vi "Xml_Get_Version.vi"(8 "error in (no error)":errorcluster, 10 "XML Path":path=path "D:/TEST.xml", 11 "Refnum Cluster":refnum<vi>) -> (0 "error out":errorcluster, 3 "Version String":string)   [LabVIEW 2020]
doc: "This VI returns the XML version of a XML file.\nIf no XML version si found, returns an empty String."
uses:
  controls/EXPERT_Inputs.ctl
  controls/DIGIT_5122_Inputs.ctl
  <instrlib>/niScope/Controls/niScope trigger source.ctl
  controls/HSDIO_6541_Inputs.ctl
  <instrlib>/niHSDIO/niHSDIO.llb/niHSDIO_ctl Trigger Source Values (Ring).ctl
  controls/SOFTWARE_Inputs.ctl
  controls/AO_6711_Inputs.ctl
  controls/AWG_5421_Inputs.ctl
  <instrlib>/niFgen/niFgen.llb/niFgen_ctl Trigger Source Values (Ring).ctl
  controls/XML_Inputs.ctl
  <vilib>/NI/GXML/GXML.lvlib
panel:
  in  "EXPERT Inputs":T1={"DIGIT 5122 Inputs"={"Sample Rate"=10000.0, "Resource Name"="DIGIT_5122", "Channel Name"="0", "Trigger Source"="VAL_EXTERNAL", "Vertical Range"=10.0, "Trigger Level"=3.0}, "HSDIO 6541 Inputs"={"Resource Name"="HSDIO_6541", "Clock Rate"=1000000.0, "Trigger Source"="PFI0"}, "SOFTWARE Inputs"={"Application Directory"=path "D:/S.O.F.T.S/LABVIEW/PIL", "Software Version"="1.0.0", "Data Path"=path "D:/PIRENEA/DATA", "XML Path"=path "D:/PIRENEA/DATA", "XML File Filter"="*.xml", "XML Saved Path"=path "D:/PIRENEA/DATA/SAVED", "Excit Scripts Path"=path "D:/PIRENEA/EXCIT_SCRIPTS", "Excit Scripts File Filter"="*.txt", "Excit Waveforms Path"=path "D:/PIRENEA/EXCIT_WFMS", "Excit Waveforms File Filter"="*.bin", "Timing Scripts Path"=path "D:/PIRENEA/TIMING_SCRIPTS", "Timing Scripts File Filter"="*.txt", "Timing Waveforms Path"=path "D:/PIRENEA/TIMING_WFMS", "Timing Waveforms File Filter"="*.bin", "Trapping Waveforms Path"=path "D:/PIRENEA/TRAPPING_WFMS", "Trapping Waveforms File Filter"="*.bin"}, "AO 6711 Inputs"={"Physical Channels"="AO_6711/ao0:3", "Min Voltage"=-10.0, "Max Voltage"=10.0, "Trigger Source"="/AO_6711/PFI3", "Counter"="AO_6711/ctr0"}, "AWG 5421 Inputs"={"Resource Name"="AWG_5421", "Sample Rate"=10000000.0, "Trigger Type"=2, "Trigger Source"="PFI0", "Waveform Gain"=0.31, "Digital Filter ON"=TRUE}, "XML Inputs"={"Version Tag Name"="XML_Version", "Version String"="1.0"}} {"AWG 5421 Inputs"."Sample Rate" format="%.2p"; "AWG 5421 Inputs"."Trigger Type" items=["None", "Software Edge", "Digital Edge", "Digital Level"]; "AO 6711 Inputs"."Max Voltage" min=-10.0 max=10.0; "AO 6711 Inputs"."Min Voltage" min=-10.0 max=10.0; "HSDIO 6541 Inputs"."Clock Rate" format="%.2p"; "DIGIT 5122 Inputs"."Trigger Level" format="%.2f"; "DIGIT 5122 Inputs"."Vertical Range" format="%.2f"; "DIGIT 5122 Inputs"."Sample Rate" step=65535.0 format="%#_3p"}
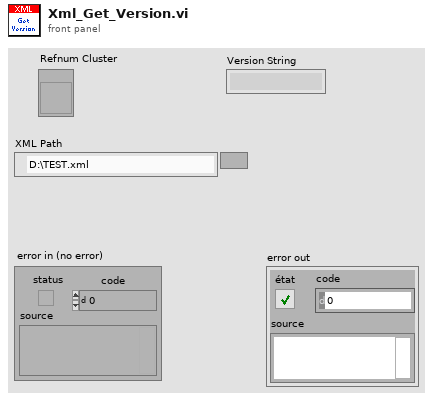
[diagram p1: front panel]
types:
  T1 = typedef "EXPERT_Inputs.ctl" = cluster{"DIGIT 5122 Inputs":T2, "HSDIO 6541 Inputs":T4, "SOFTWARE Inputs":T6, "AO 6711 Inputs":T7, "AWG 5421 Inputs":T8, "XML Inputs":T10}
  T2 = typedef "DIGIT_5122_Inputs.ctl" = cluster{"Sample Rate":dbl, "Resource Name":refnum<k15>, "Channel Name":string, "Trigger Source":T3, "Vertical Range":dbl, "Trigger Level":dbl}
  T3 = typedef "niScope trigger source.ctl" = string
  T4 = typedef "HSDIO_6541_Inputs.ctl" = cluster{"Resource Name":refnum<k15>, "Clock Rate":dbl, "Trigger Source":T5}
  T5 = typedef "niHSDIO_ctl Trigger Source Values (Ring).ctl" = string
  T6 = typedef "SOFTWARE_Inputs.ctl" = cluster{"Application Directory":path, "Software Version":string, "Data Path":path, "XML Path":path, "XML File Filter":string, "XML Saved Path":path, "Excit Scripts Path":path, "Excit Scripts File Filter":string, "Excit Waveforms Path":path, "Excit Waveforms File Filter":string, "Timing Scripts Path":path, "Timing Scripts File Filter":string, "Timing Waveforms Path":path, "Timing Waveforms File Filter":string, "Trapping Waveforms Path":path, "Trapping Waveforms File Filter":string}
  T7 = typedef "AO_6711_Inputs.ctl" = cluster{"Physical Channels":tag, "Min Voltage":dbl, "Max Voltage":dbl, "Trigger Source":tag, "Counter":tag}
  T8 = typedef "AWG_5421_Inputs.ctl" = cluster{"Resource Name":refnum<k15>, "Sample Rate":dbl, "Trigger Type":u16, "Trigger Source":T9, "Waveform Gain":dbl, "Digital Filter ON":bool}
  T9 = typedef "niFgen_ctl Trigger Source Values (Ring).ctl" = string
  T10 = typedef "XML_Inputs.ctl" = cluster{"Version Tag Name":string, "Version String":string}
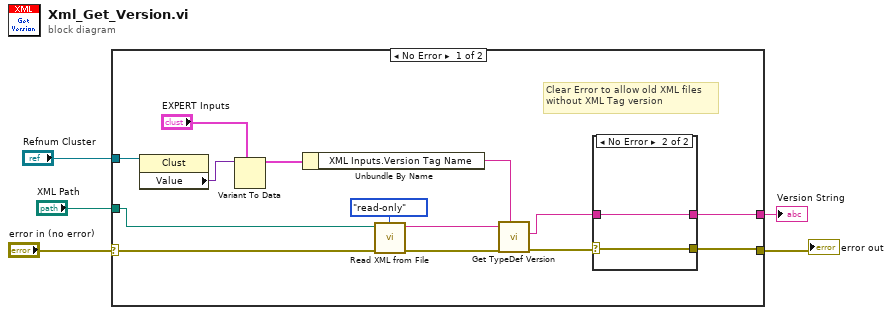
[diagram p0: block diagram]
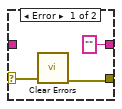
[diagram p2: hidden frame]
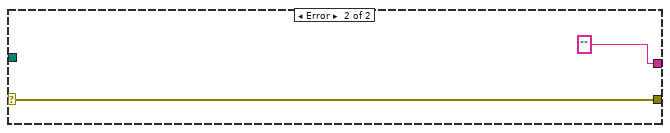
[diagram p3: hidden frame]
diagram:
  n1 = case shown="No Error" "error in (no error)" {
    selector: "error in (no error)" -> [w17 w26]
    tunnel: [w7 w26] -> w4
    tunnel: "XML Path" -> [w18 _]
    tunnel: [w16 "" ("Version String")] -> w2
    tunnel: "Refnum Cluster" -> [w14 _]
    frame No Error {
      # "Clear Error to allow old XML files\nwithout XML Tag version"
      n2 = property class="Clust"(reference=w14) -> ("Value"=w13:variant)  [unwired: 1 in, 2 out]
      n3 = Variant To Data(type="EXPERT Inputs", Variant=w13) -> (data=w19:T1)  [unwired: 1 in, 1 out]
      n4 = Unbundle By Name(w19) -> ("XML Inputs.Version Tag Name"=w11:string)
      n5 = call <vilib>:"Read XML from File.vi"("error in"=w17, "file access"=enum16{"read/write", "read-only", "write-only"}."read-only", "XML File Path"=w18) -> ("error out"=w12:errorcluster, "XML String Out"=w8:string)  [unwired: 7 in]
      n6 = call <vilib>:"Get TypeDef Version.vi"("Version Tag Name"=w11, "error in"=w12, "XML String In"=w8) -> ("error out"=w10:errorcluster, "Version String"=w9:string)  [unwired: 6 in, 1 out]
      n7 = case shown="No Error" w10 {
        selector: w10 -> [w21 w23]
        tunnel: ["" ("Version String") w24] -> w16
        tunnel: w9 -> [_ w24]
        tunnel: [w20 w23] -> w7
        frame Error {
          n8 = call <vilib>:"Clear Errors.vi"("error in (no error)"=w21) -> ("error out"=w20:errorcluster)  [unwired: 5 in, 1 out]
        }
        frame No Error {
        }
      }
    }
    frame Error {
    }
  }
  "error out" <- w4
  "Version String" <- w2
